vi "Edit Plugin Data File.vi"(0 "configuration":T1, 5 "Data File Path":path, 11 "error in":errorcluster) -> (15 "error out":errorcluster)   [LabVIEW 2021, in "InstrumentStudio Plug-In Editor.lvlib"]
uses:
  InstrumentStudio Plug-In Editor.lvlib
  Data Holder.ctl
  <vilib>/xml/Load XML String.vi
  <vilib>/xml/Close Reference(Node).vi
  <vilib>/xml/NI_XML.lvlib
  <resource>/objmgr/DOMUserDefRef.rc
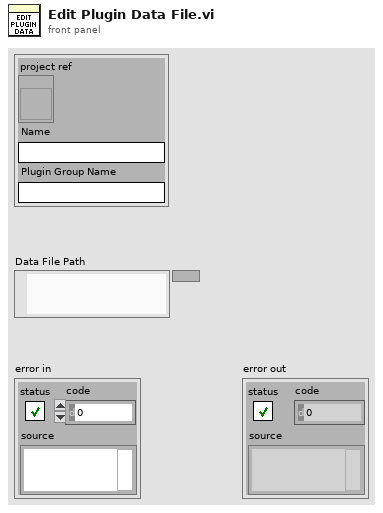
[diagram p1: front panel]
types:
  T1 = typedef "InstrumentStudio Plug-In Editor.lvlib/Data Holder.ctl" = cluster{"project ref":refnum<vi>, "Name":string, "Plugin Group Name":string}
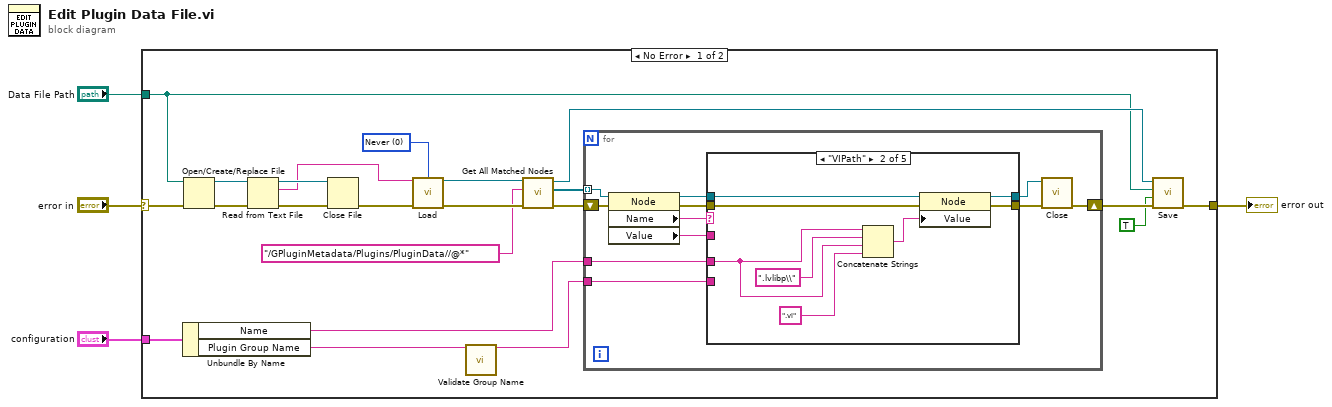
[diagram p0: block diagram]
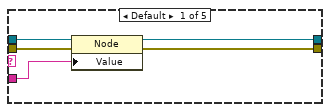
[diagram p2: hidden frame]
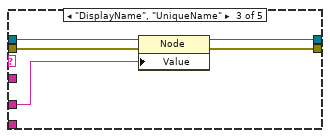
[diagram p3: hidden frame]
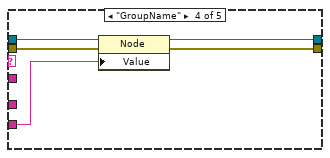
[diagram p4: hidden frame]
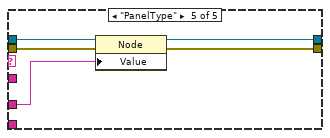
[diagram p5: hidden frame]
diagram:
  n1 = case shown="No Error" "error in" {
    selector: "error in" -> [w15 w66]
    tunnel: [w23 w66] -> w4
    tunnel: "Data File Path" -> [w11 _]
    tunnel: "configuration" -> [w22 _]
    frame No Error {
      w8 = 0 items=["Never", "Always", "Auto"] ("validate on load (Auto)")
      n2 = Unbundle By Name(w22) -> ("Name"=w21:string, "Plugin Group Name"=w7:string)
      n3 = Open/Create/Replace File(file path (use dialog)=w11, error in=w15) -> (refnum out=w26:refnum<file>, error out=w14:errorcluster)  [unwired: 4 in, 1 out]
      n4 = Read from Text File(file (use dialog)=w26, error in=w14) -> (refnum out=w25:refnum<file>, text=w9:string, error out=w13:errorcluster)  [unwired: 2 in, 1 out]
      n5 = Close File(refnum=w25, error in=w13) -> (error out=w12:errorcluster)  [unwired: 1 out]
      n6 = call-poly <vilib>:"Load.vi"("XML string"=w9, "validate on load (Auto)"=w8, "error in (no error)"=w12) -> ("DOM document out"=w10:refnum<k20>, "error out"=w18:errorcluster)  [unwired: 10 in, 1 out]
      n7 = call "Validate Group Name.vi"("Group Name in"=w7) -> ("Group Name out"=w20:string)  [unwired: 14 in]
      n8 = call <vilib>:"Get All Matched Nodes.vi"("error in (no error)"=w18, "XPath expression"="/GPluginMetadata/Plugins/PluginData//@*", "node in"=w10) -> ("error out"=w17:errorcluster, "node result array"=w19:refnum<k20>[], "node out"=w24:refnum<k20>)  [unwired: 6 in]
      n9 = for {
        tunnel: w19 -> [w37] mode=indexing
        tunnel: w21 -> [w33]
        tunnel: w20 -> [w32]
        shift-right: [w27] -> w16
        shift-left: w17 -> [w30]
        n10 = property class="Node"(reference=w37, error in=w30) -> (reference out=w36:refnum<k20>, error out=w29:errorcluster, "Name"=w34:string, "Value"=w31:string)
        n11 = case shown="\"VIPath\"" w34 {
          tunnel: w36 -> [w42 w50 w55 w60 w65]
          tunnel: [w41 w49 w54 w56 w64] -> w35
          tunnel: [w40 w46 w53 w57 w63] -> w28
          tunnel: w33 -> [_ w45 w52 _ w62]
          tunnel: w32 -> [_ _ _ w59 _]
          tunnel: w31 -> [w39 _ _ _ _]
          tunnel: w29 -> [w38 w47 w51 w58 w61]
          frame Default {
            n12 = property class="Node"(reference=w42, error in=w38, "Value"=w39) -> (reference out=w41:refnum<k20>, error out=w40:errorcluster)
          }
          frame "VIPath" {
            n13 = Concatenate Strings(w45, ".lvlibp\\" ("string"), w45, ".vi" ("string")) -> (w44:string)
            n14 = property class="Node"(reference=w50, error in=w47, "Value"=w44) -> (reference out=w49:refnum<k20>, error out=w46:errorcluster)
          }
          frame "DisplayName", "UniqueName" {
            n15 = property class="Node"(reference=w55, error in=w51, "Value"=w52) -> (reference out=w54:refnum<k20>, error out=w53:errorcluster)
          }
          frame "GroupName" {
            n16 = property class="Node"(reference=w60, error in=w58, "Value"=w59) -> (reference out=w56:refnum<k20>, error out=w57:errorcluster)
          }
          frame "PanelType" {
            n17 = property class="Node"(reference=w65, error in=w61, "Value"=w62) -> (reference out=w64:refnum<k20>, error out=w63:errorcluster)
          }
        }
        n18 = call-poly <vilib>:"Close.vi"("error in (no error)"=w28, "node"=w35) -> ("error out"=w27:errorcluster)  [unwired: 7 in]
      }
      n19 = call <vilib>:"Save.vi"("error in (no error)"=w16, "overwrite file (True)"=TRUE, "XML file path"=w11, "DOM document in"=w24) -> ("error out"=w23:errorcluster)  [unwired: 5 in, 2 out]
    }
    frame Error {
    }
  }
  "error out" <- w4
